vi "Till Array.vi"(5 "数值":u8, 7 "字节个数":i32, 11 "input":u8[](array[numeric])) -> (3 "output":u8[](array[numeric]))   [LabVIEW 2016, in "DGUS.lvlib" / "DGUS.lvclass"]
uses:
  DGUS.lvclass
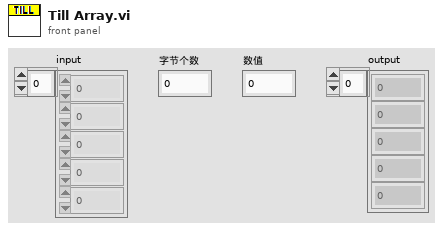
[diagram p1: front panel]
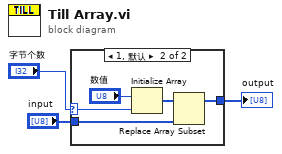
[diagram p0: block diagram]
diagram:
  n1 = case shown="1, 默认" "字节个数" {
    selector: "字节个数" -> [_ w5]
    tunnel: [w4 w7] -> w3
    tunnel: "input" -> [w4 w6]
    frame 0 {
    }
    frame 1, Default {
      n2 = Initialize Array("数值", w5) -> (w8:u8[])
      n3 = Replace Array Subset(array=w8, new element=w6) -> (w7:u8[])  [unwired: 1 in]
    }
  }
  "output" <- w3
